vi "help.vi"(10 "a fájl neve(.txt nem kell)":string, 11 "Segítség":bool) -> ()   [LabVIEW 2014]
doc: "Egy logikai TRUE értékre(pl. egy gomb megnyomására) megnyit egy txt fájlt az alkalmazás futtatási könyvtárából."
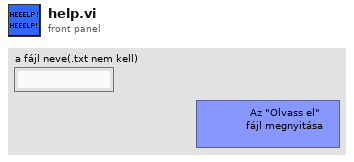
[diagram p1: front panel]
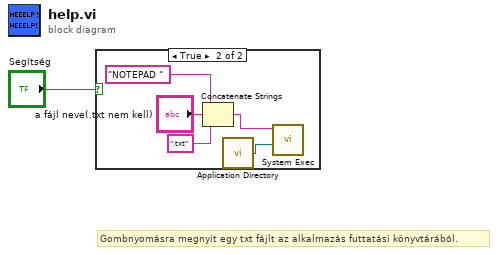
[diagram p0: block diagram]
diagram:
  # "Gombnyomásra megnyit egy txt fájlt az alkalmazás futtatási könyvtárából."
  n1 = case shown="True" "Segítség" {
    frame False {
    }
    frame True {
      n2 = Concatenate Strings("NOTEPAD " ("string"), "a fájl neve(.txt nem kell)", ".txt" ("string")) -> (w2:string)
      n3 = call <vilib>:"Application Directory.vi"() -> ("Application Directory"=w6:path)
      n4 = call <vilib>:"System Exec.vi"("working directory"=w6, "command line"=w2) -> ()  [unwired: 6 in, 4 out]
    }
  }
